vi "AlliGator Get Channel Names & Indices.vi"(8 "error in (no error)":errorcluster, 10 "# Gates":i32, 11 "File Info":variant) -> (0 "error out":errorcluster, 1 "Gate Indices":i32[](array[numeric]), 2 "Channel Arithmetic":T2, 3 "Gate Image Names":string[](array[string]), 4 "Selected Channel Name":string, 5 "Dual-Channel Dataset":bool, 6 "Selected Channel Message":string, 7 "Dataset Channel":T1)   [LabVIEW 2021, in "AlliGator Dual-Channel Datasets.lvlib"]
doc: "Returns information on the dataset file's channel(s)."
uses:
  AlliGator Dual-Channel Datasets.lvlib
  AlliGator Gate Arithmetic.ctl
  AlliGator Dataset Channel.ctl
  AlliGator FLI Dataset Type.ctl
  AlliGator HDF5 FLI File Loading Information v0.6.ctl
  AlliGator Image Folder Loading Information.ctl
  AlliGator RecSettings Metadata.ctl
  AlliGator HDF5.lvlib
  AlliGator Files.lvlib
  Files/Files.lvlib
  Image/Image.lvlib
  AlliGator Settings.lvlib
  Utilities/Utilities.lvlib
  Time/Time.lvlib
panel:
  out "Time (s)":dbl
  # "see the AlliGator License on the block diagram (Ctrl+E or Window:Show Block Diagram)"
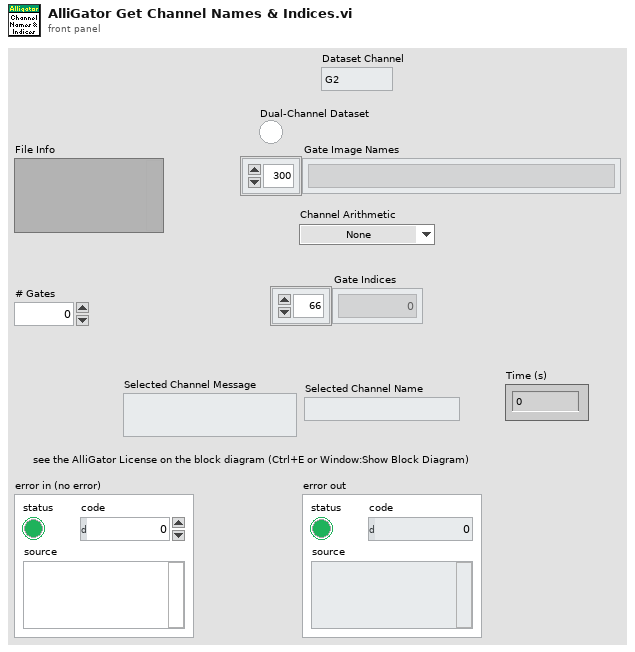
[diagram p1: front panel]
types:
  T1 = typedef "AlliGator Dual-Channel Datasets.lvlib/AlliGator Dataset Channel.ctl" = enum16{"G2", "INT"}
  T2 = typedef "AlliGator Settings.lvlib/AlliGator Gate Arithmetic.ctl" = enum16{"None", "INT-G2", "G2/INT*<INT>", "(1 - G2/INT)*<INT>"}
  T3 = typedef "AlliGator Files.lvlib/AlliGator FLI Dataset Type.ctl" = enum16{"HDF5 FLI Dataset", "Gate Image Folder", ".sdt FLI Dataset (Becker & Hickl)", ".ptu FLI Dataset (PicoQuant)", "SS1 FLI Dataset", "SS2 FLI Dataset", "I/m/phi Dataset", ".bin FLI Dataset (PicoQuant Binned)", ".bin FLI Dataset (Piccolo Binned)"}
  T4 = typedef "AlliGator HDF5.lvlib/AlliGator HDF5 FLI File Loading Information v0.6.ctl" = cluster{"HDF5 File Path":path, "Data Type":string, "# Datasets in Series":i32, "Dataset ID in Series":i32, "Channel Names":string[]}
  T5 = typedef "AlliGator Files.lvlib/AlliGator Image Folder Loading Information.ctl" = cluster{"Image Folder":path, "Metadata":T6}
  T6 = typedef "AlliGator Files.lvlib/AlliGator RecSettings Metadata.ctl" = cluster{"Time Stamp (s)":dbl, "First Gate":dbl[unit], "Gate Step":dbl[unit], "# Gates":i32, "Gate Duration":dbl[unit], "Laser Period":dbl[unit], "Gate Image Integration":dbl[unit], "Date":timestamp}
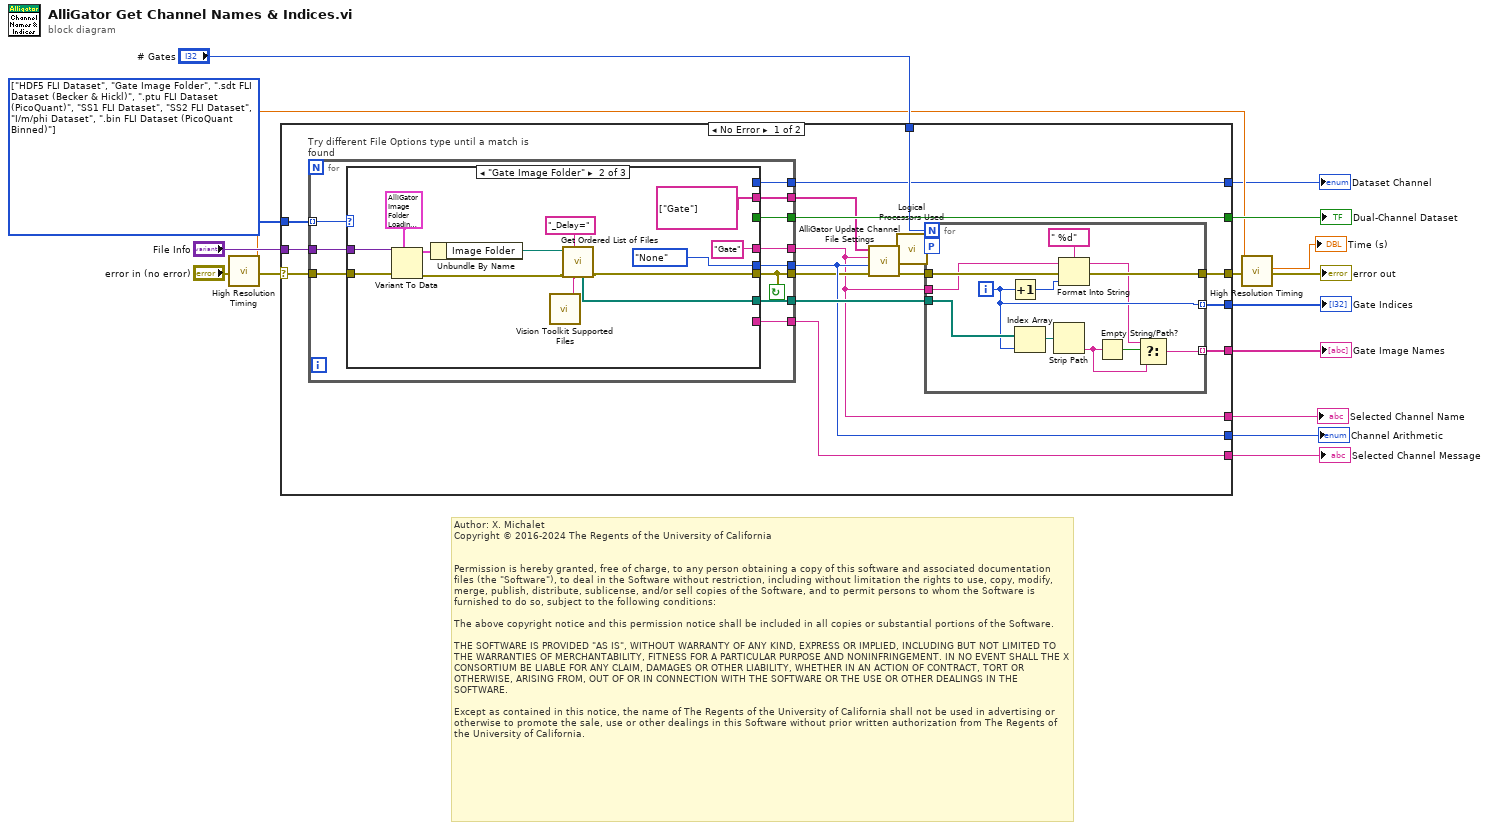
[diagram p0: block diagram]
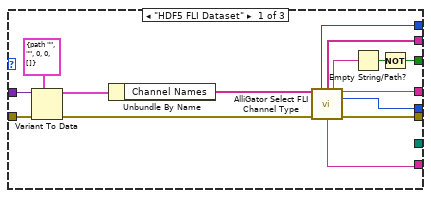
[diagram p2: hidden frame]
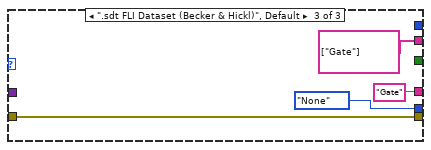
[diagram p3: hidden frame]
diagram:
  w10 = T3[] [enum."HDF5 FLI Dataset", enum."Gate Image Folder", enum.".sdt FLI Dataset (Becker & Hickl)", enum.".ptu FLI Dataset (PicoQuant)", enum."SS1 FLI Dataset", enum."SS2 FLI Dataset", enum."I/m/phi Dataset", enum.".bin FLI Dataset (PicoQuant Binned)"] items=["HDF5 FLI Dataset", "Gate Image Folder", ".sdt FLI Dataset (Becker & Hickl)", ".ptu FLI Dataset (PicoQuant)", "SS1 FLI Dataset", "SS2 FLI Dataset", "I/m/phi Dataset", ".bin FLI Dataset (PicoQuant Binned)", ".bin FLI Dataset (Piccolo Binned)"] ("Array")
  # "Author: X. Michalet\nCopyright © 2016-2024 The Regents of the University of California\n \n\nPermission is hereby granted, free of charge, to any person obtaining a copy of this software and associated documentation files (the \"Software\"), to deal in the Software without restriction, including without limitation the rights to use, copy, modify, merge, publish, distribute, sublicense, and/or sell copies of the Software, and to permit persons to whom the Software is furnished to do so, subject to the following conditions:\n\nThe above copyright notice and this permission notice shall be included in all copies or substantial portions of the Software.\n\nTHE SOFTWARE IS PROVIDED \"AS IS\", WITHOUT WARRANTY OF ANY KIND, EXPRESS OR IMPLIED, INCLUDING BUT NOT LIMITED TO THE WARRANTIES OF MERCHANTABILITY, FITNESS FOR A PARTICULAR PURPOSE AND NONINFRINGEMENT. IN NO EVENT SHALL THE X CONSORTIUM BE LIABLE FOR ANY CLAIM, DAMAGES OR OTHER LIABILITY, WHETHER IN AN ACTION OF CONTRACT, TORT OR OTHERWISE, ARISING FROM, OUT OF OR IN CONNECTION WITH THE SOFTWARE OR THE USE OR OTHER DEALINGS IN THE SOFTWARE.\n\nExcept as contained in this notice, the name of The Regents of the University of California shall not be used in advertising or otherwise to promote the sale, use or other dealings in this Software without prior written authorization from The Regents of the University of California."
  n1 = call "High Resolution Timing.vi"("Error In"="error in (no error)") -> ("elapsed (relative) seconds"=w3:dbl, "Error Out"=w5:errorcluster)  [unwired: 16 in, 1 out]
  n2 = case shown="No Error" w5 {
    selector: w5 -> [w18 w89]
    tunnel: [w33 w89] -> w16
    tunnel: "File Info" -> [w32 _]
    tunnel: "# Gates" -> [w31 _]
    tunnel: [w30 _] -> w13
    tunnel: [w29 _] -> w12
    tunnel: w10 -> [w28 _]
    tunnel: [w26 _] -> w9
    tunnel: [w25 _] -> w8
    tunnel: [w23 _] -> w7
    tunnel: [w20 _] -> w6
    tunnel: [w17 _] -> w1
    frame No Error {
      n3 = for "Try different File Options type until a match is found" {
        tunnel: [w56] -> w20
        tunnel: w32 -> [w55]
        tunnel: w28 -> [w53] mode=indexing
        tunnel: w18 -> [w54]
        tunnel: [w52] -> w22
        tunnel: [w51] -> w27
        tunnel: [w50] -> w23
        tunnel: [w49] -> w26
        tunnel: [w48] -> w25
        tunnel: [w47] -> w24
        tunnel: [w46] -> w17
        stop <- w52 continue-if-true
        n4 = case shown="\"Gate Image Folder\"" w53 {
          tunnel: [w71 w75 w87] -> w52
          tunnel: [w70 "Gate" ("Gate Name") "Gate" ("Gate Name")] -> w56
          tunnel: w55 -> [w67 w81 _]
          tunnel: w54 -> [w66 w83 w87]
          tunnel: [_ w74 _] -> w51
          tunnel: [w64 AlliGator_Gate_Arithmetic."None" ("Gate Arithmetic") AlliGator_Gate_Arithmetic."None" ("Gate Arithmetic")] -> w50
          tunnel: [w62 _ _] -> w49
          tunnel: [w60 _ _] -> w48
          tunnel: [w59 string[] ["Gate"] ("Available Gate Names") string[] ["Gate"] ("Available Gate Names")] -> w47
          tunnel: [w58 _ _] -> w46
          frame "HDF5 FLI Dataset" {
            n5 = Variant To Data(error in=w66, type=T4 {"HDF5 File Path"=path "", "Data Type"="", "# Datasets in Series"=0, "Dataset ID in Series"=0, "Channel Names"=[]} ("HDF5 FLI File Loading Information"), Variant=w67) -> (data=w69:T4, error out=w65:errorcluster)
            n6 = Unbundle By Name(w69) -> ("Channel Names"=w57:string[])
            n7 = call "AlliGator Select FLI Channel Type.vi"("Available Channel Names"=w57, "error in (no error)"=w65) -> ("Dataset Channel"=w58:T1, "Available Channel Names"=w59:string[], "Complementary Channel Name"=w61:string, "Selected Channel Name"=w70:string, "Channel Arithmetic"=w64:T2, "Selected Channel Message"=w60:string, "error out"=w71:errorcluster)  [unwired: 5 in, 2 out]
            n8 = Empty String/Path?(string/path=w61) -> (empty?=w63:bool)
            n9 = Not(x=w63) -> (.not. x?=w62:bool)
          }
          frame "Gate Image Folder" {
            n10 = Variant To Data(error in=w83, type=T5 {"Image Folder"=path "", "Metadata"={"Time Stamp (s)"=0.0, "First Gate"=0.0, "Gate Step"=0.0, "# Gates"=0, "Gate Duration"=0.0, "Laser Period"=0.0, "Gate Image Integration"=0.0, "Date"=timestamp(0 s since 1904-01-01)}} ("Image Folder Loading Information"), Variant=w81) -> (data=w80:T5, error out=w76:errorcluster)
            n11 = Unbundle By Name(w80) -> ("Image Folder"=w77:path)
            n12 = call "Vision Toolkit Supported Files.vi"() -> ("Pattern String"=w78:string)  [unwired: 7 in, 1 out]
            n13 = call "Get Ordered List of Files.vi"("pattern"=w78, "Split string"="_Delay=", "Error In"=w76, "Folder Path"=w77) -> ("Error Out"=w75:errorcluster, "Ordered File Paths"=w74:path[])  [unwired: 4 in, 2 out]
          }
          frame ".sdt FLI Dataset (Becker & Hickl)", Default {
          }
        }
      }
      n14 = call "AlliGator Update Channel File Settings.vi"("Error In"=w22, "Channel Arithmetic"=w23, "Selected Channel Name"=w20, "Available Channel Names"=w24) -> ("Error Out"=w21:errorcluster)  [unwired: 7 in]
      n15 = call "Logical Processors Used.vi"() -> ("# Logical Processor Used"=w19:i32)  [unwired: 6 in]
      n16 = for {
        N: w31 -> [_]
        tunnel: [w35] -> w29 mode=indexing
        tunnel: [w40] -> w30 mode=indexing
        tunnel: w21 -> [w45]
        tunnel: [w44] -> w33
        tunnel: w27 -> [w41]
        tunnel: w20 -> [w34]
        workers-P: w19 -> [_]
        i -> [w40]
        n17 = Increment(x=w40) -> (x+1=w42:i32)
        n18 = Index Array(array=w41, index=w40) -> (element=w39:path)
        n19 = Strip Path(path=w39) -> (name=w37:string)  [unwired: 1 out]
        n20 = Format Into String(format string=" %d", initial string=w34, error in=w45, w42) -> (resulting string=w36:string, error out=w44:errorcluster)
        n21 = Empty String/Path?(string/path=w37) -> (empty?=w38:bool)
        n22 = Select(t=w36, s=w38, f=w37) -> (s? t:f=w35:string)
      }
    }
    frame Error {
    }
  }
  "Selected Channel Message" <- w8
  "Gate Indices" <- w13
  "Gate Image Names" <- w12
  "Channel Arithmetic" <- w7
  "Dual-Channel Dataset" <- w9
  "Selected Channel Name" <- w6
  "Dataset Channel" <- w1
  n23 = call "High Resolution Timing.vi"("relative seconds (NaN)"=w3, "Error In"=w16) -> ("elapsed (relative) seconds"=→"Time (s)":dbl, "Error Out"=→"error out":errorcluster)  [unwired: 15 in, 1 out]
